vi "Merge Invalid DVR Error.vi"(8 "error in":errorcluster) -> (0 "error out":errorcluster)   [LabVIEW 2020, in "MeasurementLink Session Management V1.lvlib" / "Session Reservation.lvclass"]
uses:
  Session Reservation.lvclass
  MeasurementLink Measurement Server/Helpers/Error Strings Global Internal.vi
  Session Reservation.lvclass/Session Reservation.ctl
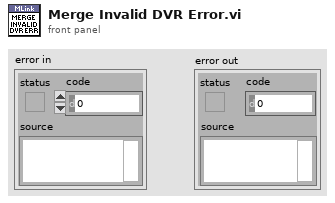
[diagram p1: front panel]
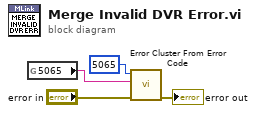
[diagram p0: block diagram]
diagram:
  n1 = global read "Error Strings Global Internal.vi" "5065"() -> (w4:string)
  n2 = call <vilib>:"Error Cluster From Error Code.vi"("error in (no error)"="error in", "error message (\"\")"=w4, "error code (0)"=5065) -> ("error out"=→"error out":errorcluster)  [unwired: 6 in]
